vi "SantecTSL210.vi"() -> ()   [LabVIEW 2019]
uses:
  Status.ctl
panel:
  out "mW":dbl
  out "nm":dbl
  out "Status":T1 {"Power (mW)" format="%.5f"; "Wavelength (nm)" format="%.5f"}
  in  "Power (mW)":sgl=-40.0 min=-40 max=20 step=0.001 format="%.3f"
  in  "Wavelength (nm)":dbl=1340.0 min=1260.0 max=1340.0 step=0.01 format="%.2f"
  in  "COH":bool
  in  "Status Cluster":T1 {"Power (mW)" format="%.5f"; "Wavelength (nm)" format="%.5f"}
  in  "LD":bool
  in  "VISA Session":refnum<visa-resource-name>
  in  "Exit":bool
  # "SANTEC TSL 210"
  # "| Control Panel"
  # "WAVELENGTH"
  # "POWER"
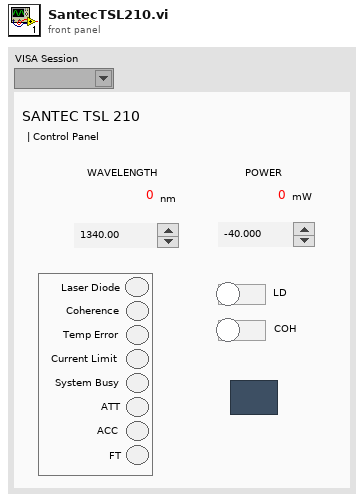
[diagram p1: front panel]
types:
  T1 = typedef "Status.ctl" = cluster{"Laser Diode":bool, "Coherence":bool, "Temp Error":bool, "Current Limit":bool, "System Busy":bool, "ATT":bool, "ACC":bool, "FT":bool, "Wavelength (nm)":ext, "Power (mW)":ext}
  T2 = enum32{"Invalid", "Standard", "Closed", "Hidden", "Minimized", "Maximized"}
  T3 = enum32{"invalid app kind", "Development System", "Run Time System", "Student Edition", "Embedded LabVIEW", "Evaluation", "Custom"}
  T4 = cluster{"Core":cluster{"Current VI Reference":refnum<vi>, "Close Panel on Exit?":bool}, "VISA Session":refnum<visa-resource-name>, "Status Cluster":T1}
  T5 = cluster{"Current VI Reference":refnum<vi>, "Close Panel on Exit?":bool}
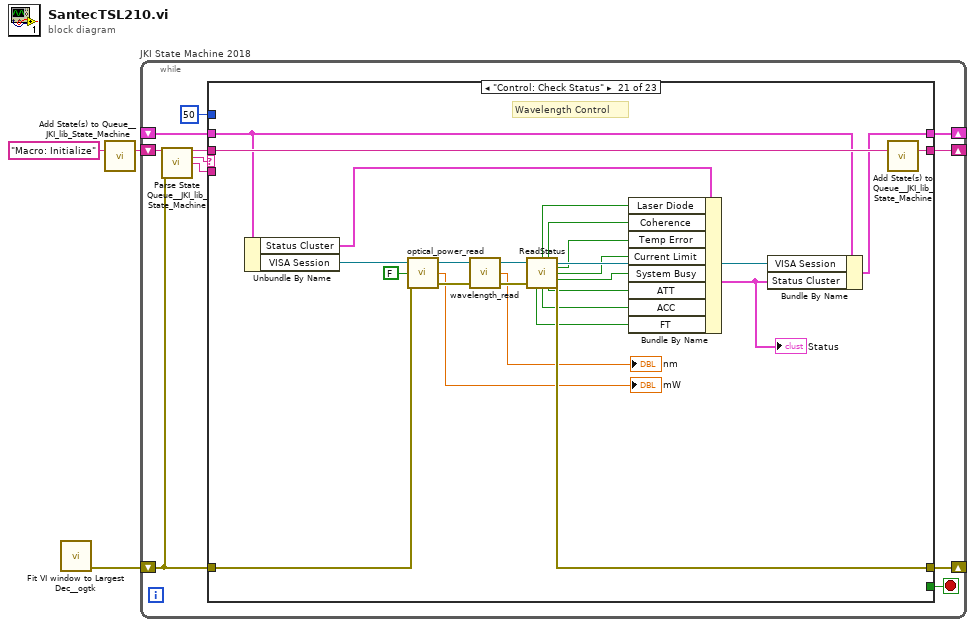
[diagram p0: block diagram]
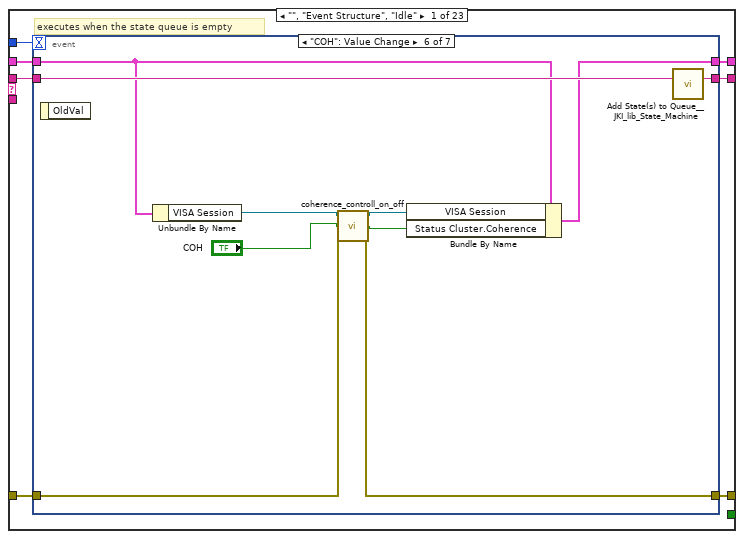
[diagram p2: hidden frame]
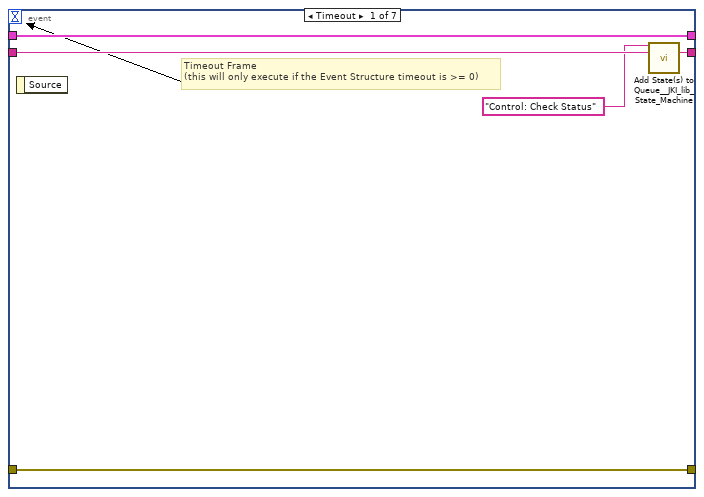
[diagram p3: hidden frame]
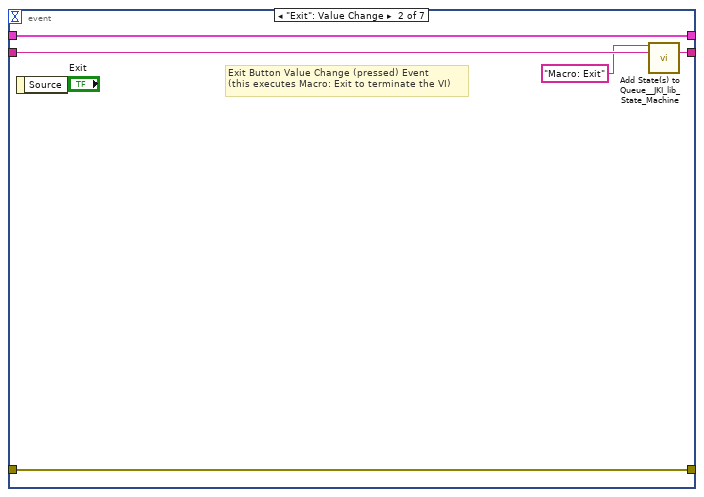
[diagram p4: hidden frame]
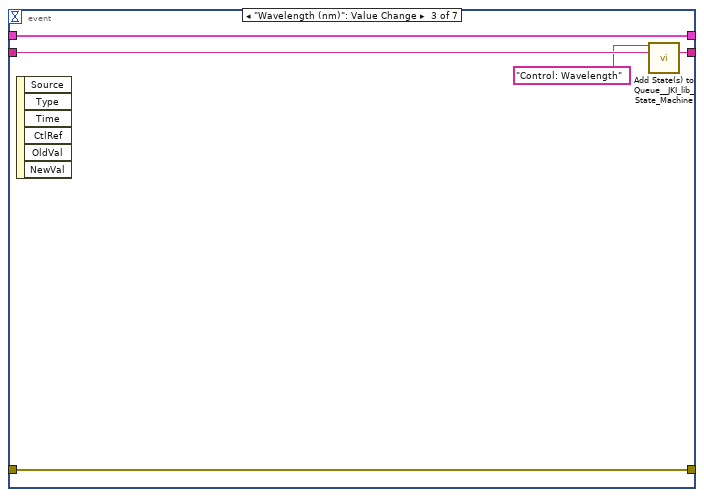
[diagram p5: hidden frame]
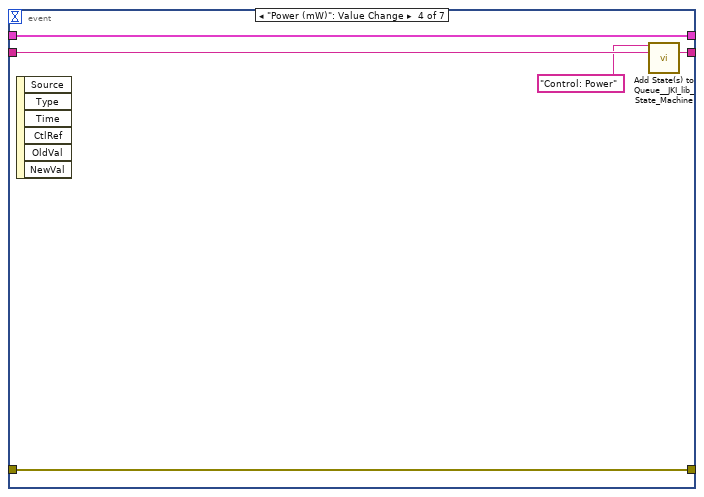
[diagram p6: hidden frame]
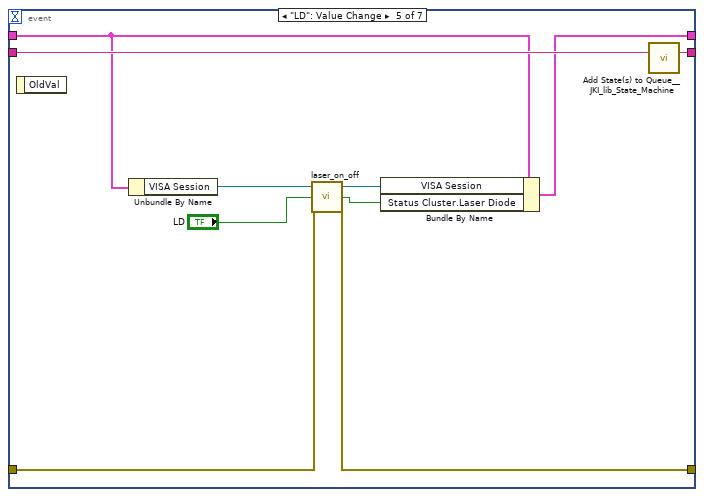
[diagram p7: hidden frame]
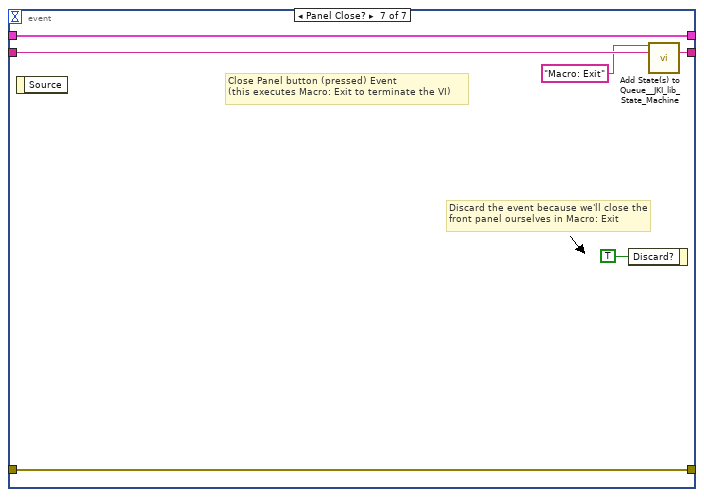
[diagram p8: hidden frame]
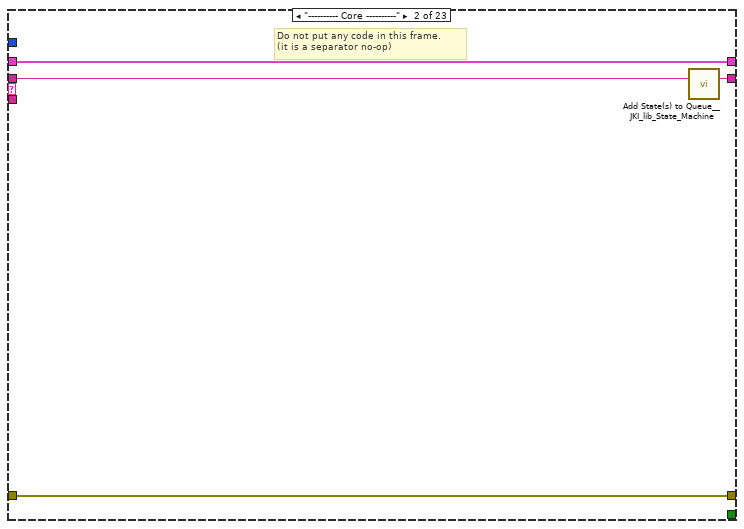
[diagram p9: hidden frame]
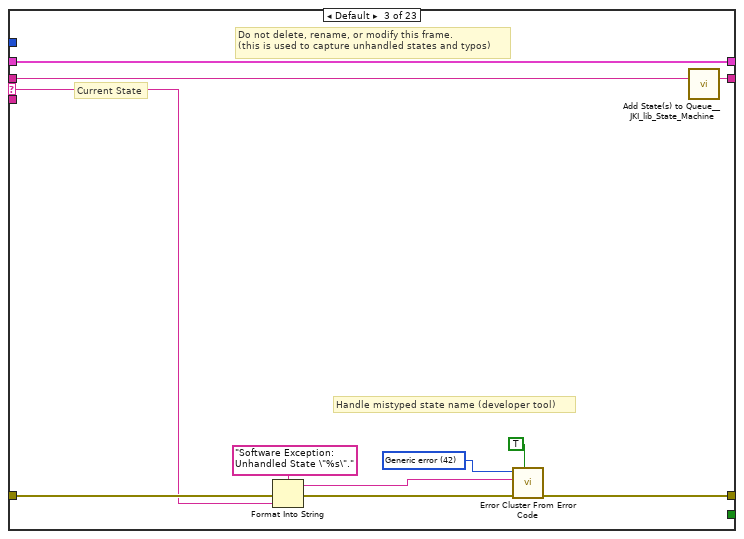
[diagram p10: hidden frame]
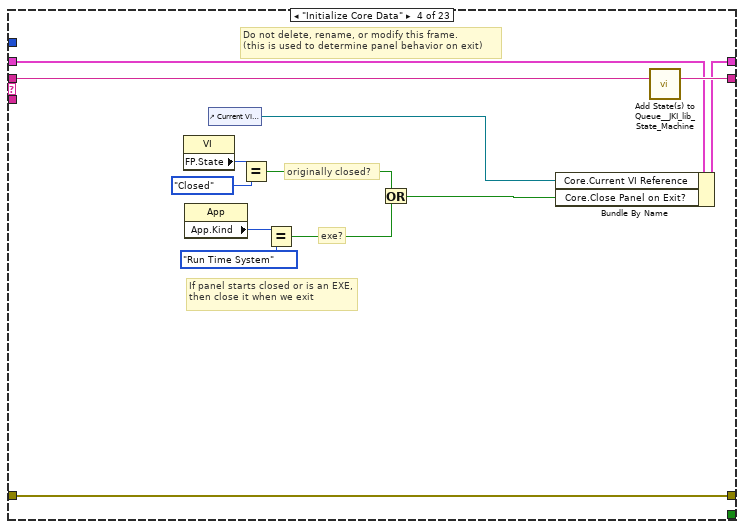
[diagram p11: hidden frame]
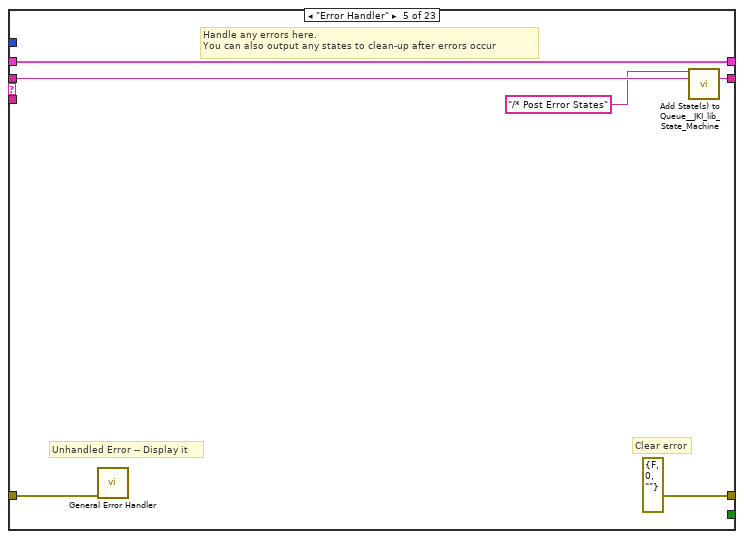
[diagram p12: hidden frame]
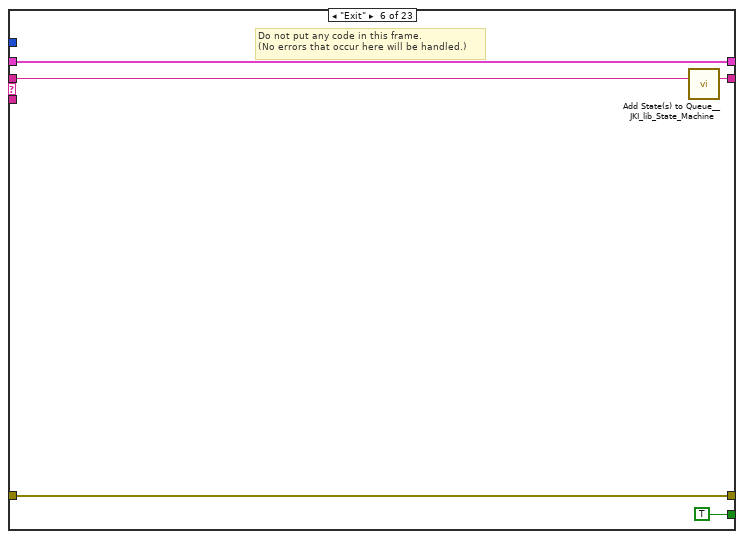
[diagram p13: hidden frame]
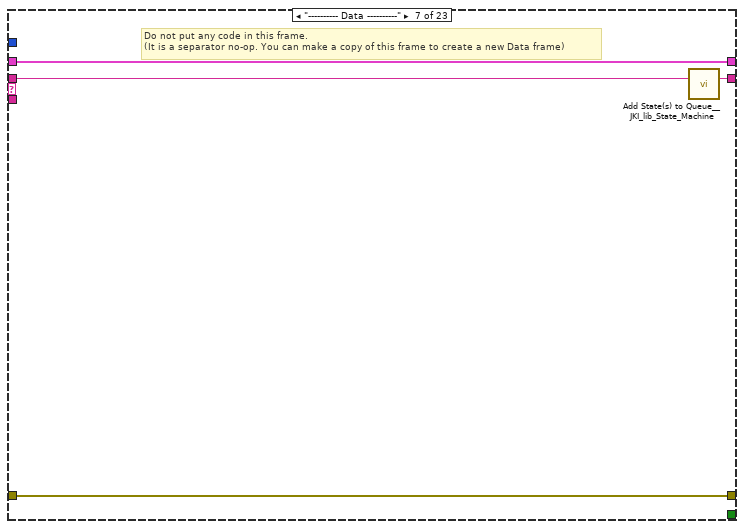
[diagram p14: hidden frame]
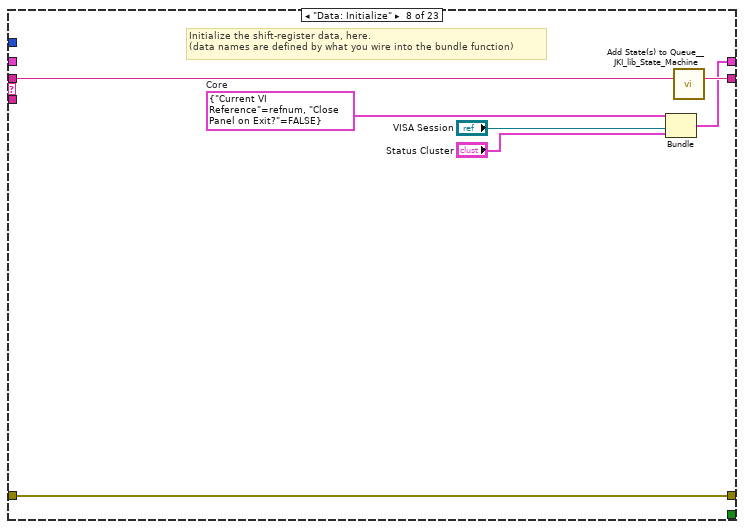
[diagram p15: hidden frame]
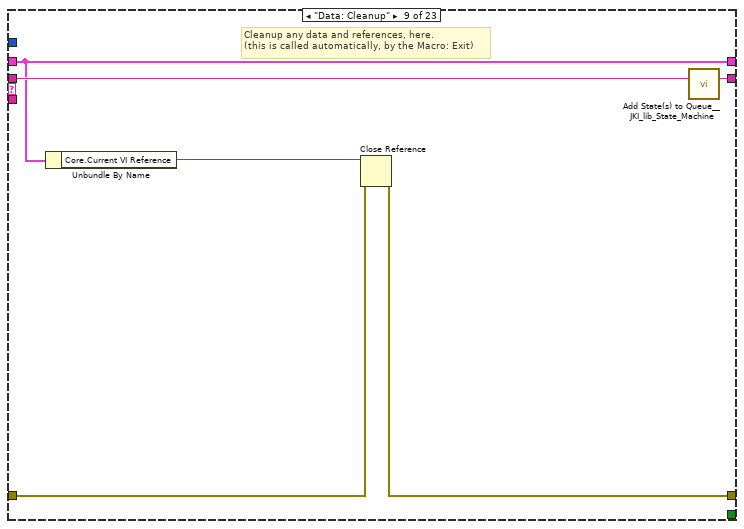
[diagram p16: hidden frame]
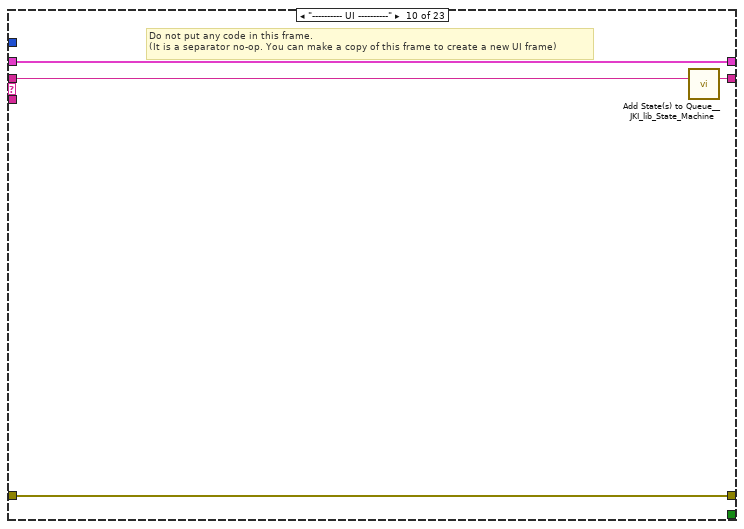
[diagram p17: hidden frame]
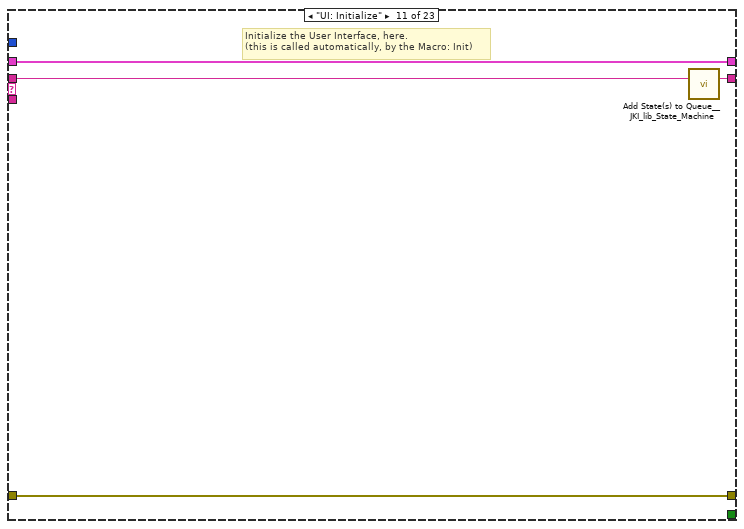
[diagram p18: hidden frame]
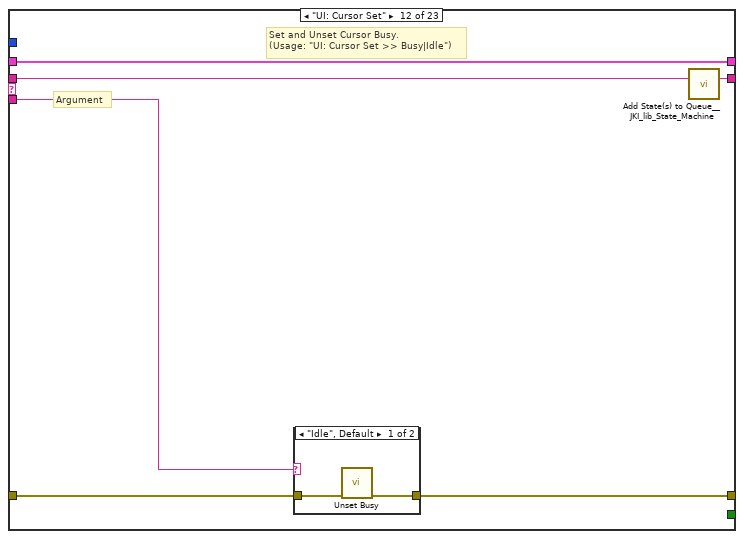
[diagram p19: hidden frame]
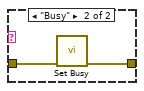
[diagram p20: hidden frame]
diagram:
  n1 = call <userlib>:"Fit VI window to Largest Dec__ogtk.vi"() -> ("error out"=w1:errorcluster)  [unwired: 6 in, 1 out]
  n2 = call <vilib>:"Add State(s) to Queue__JKI_lib_State_Machine.vi"("State(s) in (\"\")"="Macro: Initialize") -> ("States Out"=w3:string)  [unwired: 14 in]
  n3 = while "JKI State Machine 2018" {
    shift-right: [w7] -> _
    shift-left: _ -> [w6]
    shift-right: [w10] -> _
    shift-left: w1 -> [w4]
    shift-right: [w9] -> _
    shift-left: w3 -> [w11]
    stop <- w8 stop-if-true
    n4 = call <vilib>:"Parse State Queue__JKI_lib_State_Machine.vi"("State Queue"=w11, "Error In (no error)"=w4) -> ("Remaining States"=w13:string, "Current State"=w14:string, "Arguments"=w12:string)  [unwired: 11 in]
    n5 = case shown="\"Control: Check Status\"" w14 {
      selector: w14 -> [_ _ w72 _ _ _ _ _ _ _ _ _ _ _ _ _ _ _ _ _ _ _ _]
      tunnel: w13 -> [w21 w71 w76 w95 w101 w106 w110 w117 w123 w127 w131 w137 w148 w217 w222 w232 w236 w246 w252 w256 w281 w291 w302]
      tunnel: w12 -> [_ _ _ _ _ _ _ _ _ _ _ w132 w142 _ _ _ _ _ _ _ _ _ _]
      tunnel: w6 -> [w19 w68 w74 w88 w98 w104 w107 _ w118 w124 w129 w135 w144 w214 w219 w229 w233 w239 w248 w253 w279 w286 w300]
      tunnel: [w18 w69 w78 w92 errorcluster {"status"=FALSE, "code"=0, "source"=""} ("error out") w103 w108 w114 w119 w125 w128 w133 w145 w215 w220 w230 w234 w243 w249 w254 w277 w287 w297] -> w10
      tunnel: w4 -> [w17 w69 w77 w92 w97 w103 w108 w114 w120 w125 w128 w134 w146 w215 w220 w230 w234 w244 w250 w254 w273 w288 w298]
      tunnel: [w20 w70 w75 w94 w100 w105 w109 w116 w122 w126 w130 w136 w147 w216 w221 w231 w235 w245 w251 w255 w280 w290 w301] -> w9
      tunnel: [_ _ _ _ _ TRUE _ _ _ _ _ _ _ _ _ _ _ _ _ _ _ _ _] -> w8
      tunnel: [w16 w68 w74 w93 w98 w104 w107 w115 w118 w124 w129 w135 w144 w214 w219 w229 w233 w238 w248 w253 w278 w285 w299] -> w7
      tunnel: 50 ("Timeout") -> [w15 _ _ _ _ _ _ _ _ _ _ _ _ _ _ _ _ _ _ _ _ _ _]
      frame "", "Event Structure", "Idle" {
        # "executes when the state queue is empty"
        n6 = event shown="[5] \"COH\": Value Change" {
          selector: _ -> [_ _ _ _ _ _ _]
          dyn-events: _ -> [_ _ _ _ _ _ _]
          timeout: w15 -> [_ _ _ _ _ _ _]
          tunnel: w21 -> [w26 w31 w36 w41 w51 w61 w67]
          tunnel: [w25 w30 w35 w40 w50 w60 w66] -> w20
          tunnel: w19 -> [w23 w28 w33 w38 w44 w58 w64]
          tunnel: [w24 w29 w34 w39 w48 w57 w65] -> w18
          tunnel: w17 -> [w24 w29 w34 w39 w49 w56 w65]
          tunnel: [w23 w28 w33 w38 w47 w59 w64] -> w16
          event Timeout {
            # "Timeout Frame\n(this will only execute if the Event Structure timeout is >= 0)"
            n7 = event-data() -> ()  [unwired: 1 in, 1 out]
            n8 = call <vilib>:"Add State(s) to Queue__JKI_lib_State_Machine.vi"("State(s) in Front (\"\")"="Control: Check Status" ("State(s) in Front (\"\")"), "State(s) in (\"\")"=w26) -> ("States Out"=w25:string)  [unwired: 13 in]
          }
          event "Exit": Value Change {
            # "Exit Button Value Change (pressed) Event\n(this executes Macro: Exit to terminate the VI)"
            n9 = event-data() -> ()  [unwired: 1 in, 1 out]
            n10 = call <vilib>:"Add State(s) to Queue__JKI_lib_State_Machine.vi"("State(s) in Front (\"\")"="Macro: Exit", "State(s) in (\"\")"=w31) -> ("States Out"=w30:string)  [unwired: 13 in]
          }
          event "Wavelength (nm)": Value Change {
            n11 = event-data() -> ()  [unwired: 1 in, 6 out]
            n12 = call <vilib>:"Add State(s) to Queue__JKI_lib_State_Machine.vi"("State(s) in Front (\"\")"="Control: Wavelength", "State(s) in (\"\")"=w36) -> ("States Out"=w35:string)  [unwired: 13 in]
          }
          event "Power (mW)": Value Change {
            n13 = event-data() -> ()  [unwired: 1 in, 6 out]
            n14 = call <vilib>:"Add State(s) to Queue__JKI_lib_State_Machine.vi"("State(s) in Front (\"\")"="Control: Power", "State(s) in (\"\")"=w41) -> ("States Out"=w40:string)  [unwired: 13 in]
          }
          event "LD": Value Change {
            n15 = event-data() -> ()  [unwired: 1 in, 1 out]
            n16 = Unbundle By Name(w44) -> ("VISA Session"=w43:refnum<visa-resource-name>)
            n17 = call "laser_on_off.vi"("error in (no error)"=w49, "Laser ON / OFF"="LD", "VISA session (for class)"=w43) -> ("error out"=w48:errorcluster, "LD"=w46:bool, "dup VISA session"=w45:refnum<visa-resource-name>)
            n18 = Bundle By Name(cluster=w44, "VISA Session"=w45, "Status Cluster.Laser Diode"=w46) -> (w47:T4)
            n19 = call <vilib>:"Add State(s) to Queue__JKI_lib_State_Machine.vi"("State(s) in (\"\")"=w51) -> ("States Out"=w50:string)  [unwired: 14 in]
          }
          event "COH": Value Change {
            n20 = event-data() -> ()  [unwired: 1 in, 1 out]
            n21 = Unbundle By Name(w58) -> ("VISA Session"=w54:refnum<visa-resource-name>)
            n22 = call "coherence_controll_on_off.vi"("error in (no error)"=w56, "Coherence Controll\n ON / OFF"="COH", "VISA session (for class)"=w54) -> ("error out"=w57:errorcluster, "Coherence\nControl"=w52:bool, "dup VISA session"=w53:refnum<visa-resource-name>)
            n23 = Bundle By Name(cluster=w58, "VISA Session"=w53, "Status Cluster.Coherence"=w52) -> (w59:T4)
            n24 = call <vilib>:"Add State(s) to Queue__JKI_lib_State_Machine.vi"("State(s) in (\"\")"=w61) -> ("States Out"=w60:string)  [unwired: 14 in]
          }
          event Panel Close? {
            # "Discard the event because we'll close the front panel ourselves in Macro: Exit"
            # "Close Panel button (pressed) Event\n(this executes Macro: Exit to terminate the VI)"
            n25 = event-data() -> ()  [unwired: 1 in, 1 out]
            n26 = event-data("Discard?"=TRUE) -> ()  [unwired: 1 in, 1 out]
            n27 = call <vilib>:"Add State(s) to Queue__JKI_lib_State_Machine.vi"("State(s) in Front (\"\")"="Macro: Exit", "State(s) in (\"\")"=w67) -> ("States Out"=w66:string)  [unwired: 13 in]
          }
        }
      }
      frame "---------- Core ----------" {
        # "Do not put any code in this frame.\n(it is a separator no-op)"
        n28 = call <vilib>:"Add State(s) to Queue__JKI_lib_State_Machine.vi"("State(s) in (\"\")"=w71) -> ("States Out"=w70:string)  [unwired: 14 in]
      }
      frame Default {
        w81 = 42 items=["No error", "Argument error", "Memory is full", "Out of zone", "End of file", "File already open", "Generic file I/O error", "File not found", "File permission error", "Disk is full", "Duplicate path", "Too many files open", "System feature not enabled", "Resource file not found", "Cannot add resource", "Resource not found", "Image not found", "Image memory error", "Pen does not exist", "Config type invalid", "Config token not found", "Config parse error", "Config memory error", "Bad external code format", "Bad external code offset", "External code not present", "Null window", "Destroy window error", "Null menu", "Print aborted", "Bad print record", "Print driver error", "Windows error during printing", "Memory error during printing", "Print dialog error", "Generic print error", "Invalid device refnum", "Device not found", "Device parameter error", "Device unit error", "Cannot open device", "Device call aborted", "Generic error", "Cancelled by user", "Object ID too low", "Object ID too high", "Object not in heap", "Unknown heap", "Unknown object (invalid DefProc)", "Unknown object (DefProc not in table)", "Message out of range", "Invalid (null) method", "Unknown message", "Manager call not supported", "Bad address", "Network operation in progress", "Network operation timed out", "Connection is busy", "Network attribute not supported", "Network error", "Address in use", "System out of memory", "Connection aborted", "Connection refused", "Not connected", "Already connected", "Connection closed", "Initialization error (interapplication manager)", "Bad occurrence", "Wait on unbound occurrence handler", "Occurrence queue overflow", "Datalog type conflict", "Unused", "Unrecognized type (interapplication manager)", "Memory corrupt", "Failed to make temporary DLL", "Old CIN version", "Drag socket not found", "Failed to load drop-object", "Failed to register OLE object", "Failed to release OLE object", "Format specifier type mismatch", "Unknown format specifier", "Too few format specifiers", "Too many format specifiers", "Scan failed", "Newer CIN version", "Error converting to variant", "Runtime menu error", "Password tampered", "Variant attribute not found", "Incompatible variant data type", "Event data is not available", "Event Store is not present", "Occurrence is not found", "Event Queue is not created", "Event info is not available", "Refnum passed is NULL", "Error retrieving Class GUID", "Error retrieving CoClass GUID", "Error retrieving TypeLib GUID.", "Bad built application magic bytes.", "Specific driver is different from the specific driver associated with the Logical Name.", "There is no session opened to the class driver.", "Max Error", "MAX - Error with config objects", "MAX - Error loading configuration", "MAX - Group not supported"]
        # "Current State"
        # "Do not delete, rename, or modify this frame.\n(this is used to capture unhandled states and typos)"
        # "Handle mistyped state name (developer tool)"
        n29 = Format Into String(format string="Software Exception: Unhandled State \"%s\"." ("message"), error in=w77, w72) -> (resulting string=w80:string, error out=w79:errorcluster)  [unwired: 1 in]
        n30 = call <vilib>:"Error Cluster From Error Code.vi"("show call chain? (False)"=TRUE, "error in (no error)"=w79, "error message (\"\")"=w80, "error code (0)"=w81) -> ("error out"=w78:errorcluster)  [unwired: 5 in]
        n31 = call <vilib>:"Add State(s) to Queue__JKI_lib_State_Machine.vi"("State(s) in (\"\")"=w76) -> ("States Out"=w75:string)  [unwired: 14 in]
      }
      frame "Initialize Core Data" {
        # "Do not delete, rename, or modify this frame.\n(this is used to determine panel behavior on exit)"
        # "originally closed?"
        # "exe?"
        # "If panel starts closed or is an EXE, then close it when we exit"
        n32 = property class="VI"() -> ("FP.State"=w85:T2)  [unwired: 2 in, 2 out]
        n33 = property class="App"() -> ("App.Kind"=w91:T3)  [unwired: 2 in, 2 out]
        n34 = control-ref of="Current VI Reference"() -> (w86:refnum<vi>)
        n35 = Equal?(x=w85, y=T2."Closed" ("Front Panel Window:State")) -> (x = y?=w83:bool)
        n36 = Equal?(x=w91, y=T3."Run Time System" ("Application:Kind")) -> (x = y?=w89:bool)
        n37 = Or(x=w83, y=w89) -> (x .or. y?=w87:bool)
        n38 = Bundle By Name(cluster=w88, "Core.Current VI Reference"=w86, "Core.Close Panel on Exit?"=w87) -> (w93:T4)
        n39 = call <vilib>:"Add State(s) to Queue__JKI_lib_State_Machine.vi"("State(s) in (\"\")"=w95) -> ("States Out"=w94:string)  [unwired: 14 in]
      }
      frame "Error Handler" {
        # "Unhandled Error -- Display it"
        # "Handle any errors here.\nYou can also output any states to clean-up after errors occur"
        # "Clear error"
        n40 = call <vilib>:"General Error Handler.vi"("error in (no error)"=w97) -> ()  [unwired: 10 in, 5 out]
        n41 = call <vilib>:"Add State(s) to Queue__JKI_lib_State_Machine.vi"("State(s) in Front (\"\")"="/* Post Error States", "State(s) in (\"\")"=w101) -> ("States Out"=w100:string)  [unwired: 13 in]
      }
      frame "Exit" {
        # "Do not put any code in this frame.\n(No errors that occur here will be handled.)"
        n42 = call <vilib>:"Add State(s) to Queue__JKI_lib_State_Machine.vi"("State(s) in (\"\")"=w106) -> ("States Out"=w105:string)  [unwired: 14 in]
      }
      frame "---------- Data ----------" {
        # "Do not put any code in this frame.\n(It is a separator no-op. You can make a copy of this frame to create a new Data frame)"
        n43 = call <vilib>:"Add State(s) to Queue__JKI_lib_State_Machine.vi"("State(s) in (\"\")"=w110) -> ("States Out"=w109:string)  [unwired: 14 in]
      }
      frame "Data: Initialize" {
        w113 = T5 {"Current VI Reference"=refnum, "Close Panel on Exit?"=FALSE}  # Core
        # "Initialize the shift-register data, here.\n(data names are defined by what you wire into the bundle function)"
        n44 = Bundle("Core"=w113, "VISA Session"="VISA Session", "Status Cluster"="Status Cluster") -> (w115:T4)  [unwired: 1 in]
        n45 = call <vilib>:"Add State(s) to Queue__JKI_lib_State_Machine.vi"("State(s) in (\"\")"=w117) -> ("States Out"=w116:string)  [unwired: 14 in]
      }
      frame "Data: Cleanup" {
        # "Cleanup any data and references, here.\n(this is called automatically, by the Macro: Exit)"
        n46 = Unbundle By Name(w118) -> ("Core.Current VI Reference"=w121:refnum<vi>)
        n47 = Close Reference(reference=w121, error in (no error)=w120) -> (error out=w119:errorcluster)
        n48 = call <vilib>:"Add State(s) to Queue__JKI_lib_State_Machine.vi"("State(s) in (\"\")"=w123) -> ("States Out"=w122:string)  [unwired: 14 in]
      }
      frame "---------- UI ----------" {
        # "Do not put any code in this frame.\n(It is a separator no-op. You can make a copy of this frame to create a new UI frame)"
        n49 = call <vilib>:"Add State(s) to Queue__JKI_lib_State_Machine.vi"("State(s) in (\"\")"=w127) -> ("States Out"=w126:string)  [unwired: 14 in]
      }
      frame "UI: Initialize" {
        # "Initialize the User Interface, here.\n(this is called automatically, by the Macro: Init)"
        n50 = call <vilib>:"Add State(s) to Queue__JKI_lib_State_Machine.vi"("State(s) in (\"\")"=w131) -> ("States Out"=w130:string)  [unwired: 14 in]
      }
      frame "UI: Cursor Set" {
        # "Argument"
        # "Set and Unset Cursor Busy.\n(Usage: \"UI: Cursor Set >> Busy|Idle\")"
        n51 = case shown="\"Idle\", Default" w132 {
          tunnel: w134 -> [w139 w141]
          tunnel: [w138 w140] -> w133
          frame "Idle", Default {
            n52 = call <vilib>:"Unset Busy.vi"("error in (no error)"=w139) -> ("error out"=w138:errorcluster)  [unwired: 10 in]
          }
          frame "Busy" {
            n53 = call <vilib>:"Set Busy.vi"("error in (no error)"=w141) -> ("error out"=w140:errorcluster)  [unwired: 9 in, 1 out]
          }
        }
        n54 = call <vilib>:"Add State(s) to Queue__JKI_lib_State_Machine.vi"("State(s) in (\"\")"=w137) -> ("States Out"=w136:string)  [unwired: 14 in]
      }
      frame "UI: Front Panel State" {
        # "Argument"
        # "Set Front Panel Open or Closed\n(Usage: \"UI: Front Panel State >> Open|Close\")"
        n55 = Unbundle By Name(w144) -> ("Core.Current VI Reference"=w143:refnum<vi>)
        n56 = case shown="\"Minimize\", \"Minimized\"" w142 {
          tunnel: w146 -> [w154 w169 w180 w193 w206]
          tunnel: [w156 w170 w182 w195 w208] -> w145
          tunnel: w143 -> [w155 w167 w181 w194 w207]
          frame "Open", "Standard", Default {
            w149 = T2."Standard" ("State")
            n57 = property class="VI"(reference=w155, error in=w154) -> (reference out=w152:refnum<vi>, error out=w153:errorcluster, "FP.State"=w151:T2)
            n58 = Not Equal?(x=w151, y=w149) -> (x != y?=w150:bool)
            n59 = case shown="True" w150 {
              tunnel: [w160 w162] -> w156
              tunnel: w153 -> [w159 w162]
              tunnel: w152 -> [w158 _]
              tunnel: w149 -> [w157 _]
              frame True {
                n60 = invoke class="VI" method="FP.Open"(reference=w158, error in=w159, "Activate"=TRUE, "State"=w157) -> (error out=w160:errorcluster)  [unwired: 1 in, 4 out]
              }
              frame False {
              }
            }
          }
          frame "Close", "Closed" {
            n61 = property class="VI"(reference=w167, error in=w169) -> (reference out=w166:refnum<vi>, error out=w168:errorcluster, "FP.State"=w164:T2)
            n62 = Not Equal?(x=w164, y=T2."Closed" ("Front Panel Window:State")) -> (x != y?=w163:bool)
            n63 = case shown="True" w163 {
              tunnel: [w171 w174] -> w170
              tunnel: w168 -> [w171 w173]
              tunnel: w166 -> [_ w172]
              frame False {
              }
              frame True {
                n64 = invoke class="VI" method="FP.Close"(reference=w172, error in=w173) -> (error out=w174:errorcluster)  [unwired: 1 in, 2 out]
              }
            }
          }
          frame "Hidden", "Hide" {
            w175 = T2."Hidden" ("State")
            n65 = property class="VI"(reference=w181, error in=w180) -> (reference out=w178:refnum<vi>, error out=w179:errorcluster, "FP.State"=w177:T2)
            n66 = Not Equal?(x=w177, y=w175) -> (x != y?=w176:bool)
            n67 = case shown="True" w176 {
              tunnel: [w186 w187] -> w182
              tunnel: w179 -> [w185 w187]
              tunnel: w178 -> [w184 _]
              tunnel: w175 -> [w183 _]
              frame True {
                n68 = invoke class="VI" method="FP.Open"(reference=w184, error in=w185, "State"=w183) -> (error out=w186:errorcluster)  [unwired: 2 in, 4 out]
              }
              frame False {
              }
            }
          }
          frame "Minimize", "Minimized" {
            w188 = T2."Minimized" ("State")
            n69 = property class="VI"(reference=w194, error in=w193) -> (reference out=w191:refnum<vi>, error out=w192:errorcluster, "FP.State"=w190:T2)
            n70 = Not Equal?(x=w190, y=w188) -> (x != y?=w189:bool)
            n71 = case shown="True" w189 {
              tunnel: [w199 w200] -> w195
              tunnel: w192 -> [w198 w200]
              tunnel: w191 -> [w197 _]
              tunnel: w188 -> [w196 _]
              frame True {
                n72 = invoke class="VI" method="FP.Open"(reference=w197, error in=w198, "State"=w196) -> (error out=w199:errorcluster)  [unwired: 2 in, 4 out]
              }
              frame False {
              }
            }
          }
          frame "Maximize", "Maximized" {
            w201 = T2."Maximized" ("State")
            n73 = property class="VI"(reference=w207, error in=w206) -> (reference out=w204:refnum<vi>, error out=w205:errorcluster, "FP.State"=w203:T2)
            n74 = Not Equal?(x=w203, y=w201) -> (x != y?=w202:bool)
            n75 = case shown="True" w202 {
              tunnel: [w212 w213] -> w208
              tunnel: w205 -> [w211 w213]
              tunnel: w204 -> [w210 _]
              tunnel: w201 -> [w209 _]
              frame True {
                n76 = invoke class="VI" method="FP.Open"(reference=w210, error in=w211, "State"=w209) -> (error out=w212:errorcluster)  [unwired: 2 in, 4 out]
              }
              frame False {
              }
            }
          }
        }
        n77 = call <vilib>:"Add State(s) to Queue__JKI_lib_State_Machine.vi"("State(s) in (\"\")"=w148) -> ("States Out"=w147:string)  [unwired: 14 in]
      }
      frame "---------- Macro ----------" {
        # "Do not put any code in this frame.\n(It is a separator no-op. You can make a copy of this frame to create a new Macro frame)"
        n78 = call <vilib>:"Add State(s) to Queue__JKI_lib_State_Machine.vi"("State(s) in (\"\")"=w217) -> ("States Out"=w216:string)  [unwired: 14 in]
      }
      frame "Macro: Initialize" {
        w218 = "Data: Initialize\nInitialize Core Data\nUI: Initialize\nUI: Front Panel State >> Open\nHardware: Init"  # Data: Initialize Initialize Core Data UI: Initialize UI: Front Panel State >> Open Hardware: Init
        # "Initialization Macro\n(This is called once, when the VI starts)"
        n79 = call <vilib>:"Add State(s) to Queue__JKI_lib_State_Machine.vi"("State(s) in Front (\"\")"=w218, "State(s) in (\"\")"=w222) -> ("States Out"=w221:string)  [unwired: 13 in]
      }
      frame "Macro: Exit" {
        # "Exit Macro\n(This is called once, when the VI exits)"
        n80 = Unbundle By Name(w229) -> ("Core.Close Panel on Exit?"=w228:bool)
        n81 = Select(t="UI: Front Panel State >> Close", s=w228, f="") -> (s? t:f=w225:string)
        n82 = call <vilib>:"Add State(s) to Queue__JKI_lib_State_Machine.vi"("State(s) in (\"\")"=w225, "State(s) at Back (\"\")"="Hardware: Close\nData: Cleanup\nExit") -> ("States Out"=w223:string)  [unwired: 13 in]
        n83 = call <vilib>:"Add State(s) to Queue__JKI_lib_State_Machine.vi"("State(s) in Front (\"\")"=w223, "State(s) in (\"\")"=w232) -> ("States Out"=w231:string)  [unwired: 13 in]
      }
      frame "---------- Hardware ----------" {
        # "Template Separator\n(You can make a copy of, or modify, this frame)"
        n84 = call <vilib>:"Add State(s) to Queue__JKI_lib_State_Machine.vi"("State(s) in (\"\")"=w236) -> ("States Out"=w235:string)  [unwired: 14 in]
      }
      frame "Hardware: Init" {
        # "Hardware Initialization"
        n85 = call "TSL-210 Initialize.vi"("error in (no error)"=w244, "Termination Charactor"=3, "Reset (T: yes)"=FALSE, "GPIB address default: 5"=i16 1) -> ("error out"=w243:errorcluster, "dup VISA session"=w237:refnum<visa-resource-name>)  [unwired: 1 out]
        n86 = Bundle By Name(cluster=w239, "VISA Session"=w237) -> (w238:T4)
        n87 = call <vilib>:"Add State(s) to Queue__JKI_lib_State_Machine.vi"("State(s) in (\"\")"=w246) -> ("States Out"=w245:string)  [unwired: 14 in]
      }
      frame "Hardware: Close" {
        # "Hardware Closure"
        n88 = Unbundle By Name(w248) -> ("VISA Session"=w247:refnum<visa-resource-name>)
        n89 = call "TSL-210 Close.vi"("error in (no error)"=w250, "VISA Session"=w247) -> ("error out"=w249:errorcluster)
        n90 = call <vilib>:"Add State(s) to Queue__JKI_lib_State_Machine.vi"("State(s) in (\"\")"=w252) -> ("States Out"=w251:string)  [unwired: 14 in]
      }
      frame "---------- Control ----------" {
        # "Template Separator\n(You can make a copy of, or modify, this frame)"
        n91 = call <vilib>:"Add State(s) to Queue__JKI_lib_State_Machine.vi"("State(s) in (\"\")"=w256) -> ("States Out"=w255:string)  [unwired: 14 in]
      }
      frame "Control: Check Status" {
        # "Wavelength Control"
        n92 = Unbundle By Name(w279) -> ("Status Cluster"=w268:T1, "VISA Session"=w269:refnum<visa-resource-name>)
        n93 = call "optical_power_read.vi"("error in (no error)"=w273, "unit"=FALSE, "VISA session (for class)"=w269) -> ("error out"=w275:errorcluster, "optical power"=→"mW":dbl, "dup VISA session"=w272:refnum<visa-resource-name>)
        n94 = call "wavelength_read.vi"("VISA session (for class)"=w272, "error in (no error)"=w275) -> ("dup VISA session"=w271:refnum<visa-resource-name>, "wavelength in nm (numerical output)"=→"nm":ext, "error out"=w274:errorcluster)
        n95 = call "ReadStatus.vi"("VISA session"=w271, "error in (no error)"=w274) -> ("LD ON"=w267:bool, "COH"=w266:bool, "dup VISA session"=w276:refnum<visa-resource-name>, "Temp. Err."=w265:bool, "Current Limit"=w264:bool, "Busy"=w263:bool, "FT"=w260:bool, "ACC"=w261:bool, "ATT"=w262:bool, "error out"=w277:errorcluster)  [unwired: 3 in, 1 out]
        n96 = Bundle By Name(cluster=w268, "Laser Diode"=w267, "Coherence"=w266, "Temp Error"=w265, "Current Limit"=w264, "System Busy"=w263, "ATT"=w262, "ACC"=w261, "FT"=w260) -> (w259:T1)
        "Status" <- w259
        n97 = Bundle By Name(cluster=w279, "VISA Session"=w276, "Status Cluster"=w259) -> (w278:T4)
        n98 = call <vilib>:"Add State(s) to Queue__JKI_lib_State_Machine.vi"("State(s) in (\"\")"=w281) -> ("States Out"=w280:string)  [unwired: 14 in]
      }
      frame "Control: Wavelength" {
        # "Wavelength Control"
        n99 = Unbundle By Name(w286) -> ("VISA Session"=w289:refnum<visa-resource-name>)
        n100 = call "wavelength_set.vi"("error in (no error)"=w288, "Wavelength in nm"="Wavelength (nm)", "VISA session (for class)"=w289) -> ("error out"=w287:errorcluster, "wavelength in nm (numerical output)"=w283:ext, "dup VISA session"=w284:refnum<visa-resource-name>)
        n101 = Bundle By Name(cluster=w286, "VISA Session"=w284, "Status Cluster.Wavelength (nm)"=w283) -> (w285:T4)
        n102 = call <vilib>:"Add State(s) to Queue__JKI_lib_State_Machine.vi"("State(s) in (\"\")"=w291) -> ("States Out"=w290:string)  [unwired: 14 in]
      }
      frame "Control: Power" {
        # "Wavelength Control"
        n103 = Unbundle By Name(w300) -> ("VISA Session"=w295:refnum<visa-resource-name>)
        n104 = call "optical_power_set.vi"("error in (no error)"=w298, "unit dBM: TRUE\n        mW: FALSE"=FALSE ("unit dBM: TRUE\n        mW: FALSE"), "optical output power in UNIT"="Power (mW)", "VISA session (for class)"=w295) -> ("error out"=w297:errorcluster, "optical power"=w293:dbl, "dup VISA session"=w296:refnum<visa-resource-name>)
        n105 = Bundle By Name(cluster=w300, "VISA Session"=w296, "Status Cluster.Power (mW)"=w293) -> (w299:T4)
        n106 = call <vilib>:"Add State(s) to Queue__JKI_lib_State_Machine.vi"("State(s) in (\"\")"=w302) -> ("States Out"=w301:string)  [unwired: 14 in]
      }
    }
  }
